vi "PerisPump_queue_single.vi"(8 "Step":string="500", 9 "Time/min":i32, 10 "First step":enum16{"forward", "backward"}(ring), 11 "Address":u8=1) -> (2 "status":dbl(slide) scale=0.0..100.0)   [LabVIEW 2023]
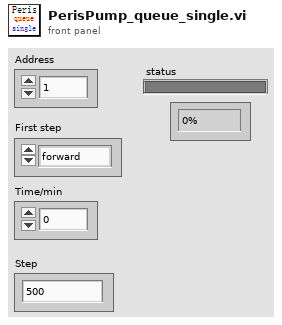
[diagram p1: front panel]
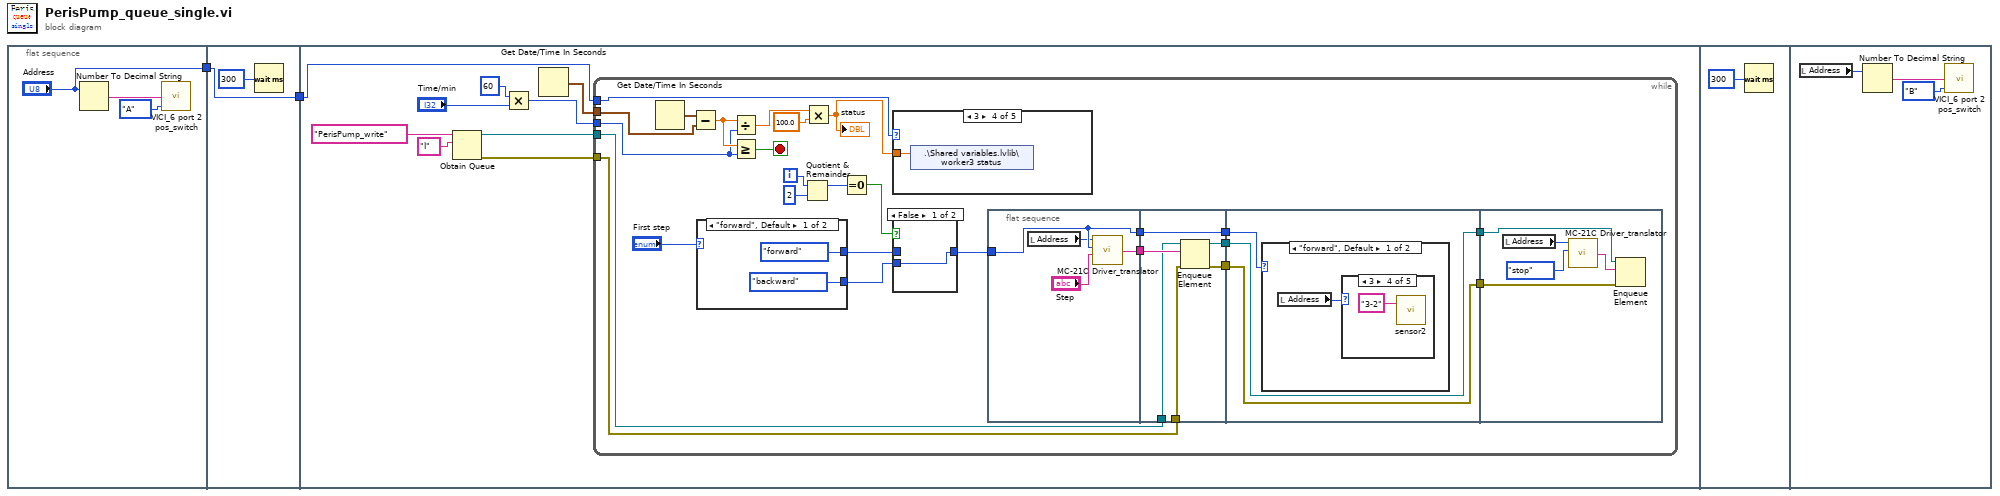
[diagram p0: block diagram]
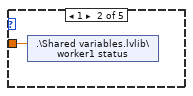
[diagram p3: hidden frame]
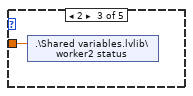
[diagram p4: hidden frame]
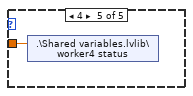
[diagram p5: hidden frame]
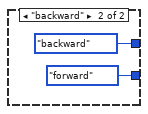
[diagram p6: hidden frame]
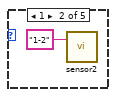
[diagram p9: hidden frame]
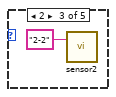
[diagram p10: hidden frame]
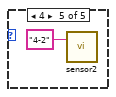
[diagram p11: hidden frame]
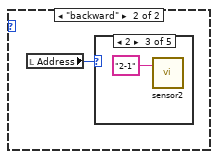
[diagram p12: hidden frame]
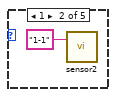
[diagram p14: hidden frame]
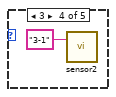
[diagram p15: hidden frame]
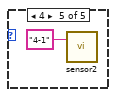
[diagram p16: hidden frame]
diagram:
  n1 = flat-sequence {
    tunnel: ["Address"] -> w1
    tunnel: [w6] -> w2
    tunnel: w1 -> [w6]
    tunnel: w2 -> [w12]
    frame #0 {
      n2 = Number To Decimal String(number="Address") -> (decimal integer string=w4:string)  [unwired: 1 in]
      n3 = call "VICI_6 port 2 pos_switch.vi"("Switch to position (A/B)"=enum16{"A", "B"}."A", "Valve ID"=w4) -> ()  [unwired: 2 in, 1 out]
    }
    frame #1 {
      n4 = Wait (ms)(milliseconds to wait=u32 300) -> ()  [unwired: 1 out]
    }
    frame #2 {
      n5 = Obtain Queue(name (unnamed)="PerisPump_write", element data type="Ì" ("string")) -> (queue out=w14:refnum<queue>, error out=w13:errorcluster)  [unwired: 3 in, 1 out]
      n6 = Multiply(x=60 ("value"), y="Time/min") -> (x*y=w8:i32)
      n7 = Get Date/Time In Seconds() -> (seconds since 1Jan1904=w11:timestamp)
      n8 = while {
        tunnel: w14 -> [w41]
        tunnel: w13 -> [w40]
        tunnel: w12 -> [w26]
        tunnel: w11 -> [w20]
        tunnel: w8 -> [w17]
        i -> [w22]
        stop <- w19 stop-if-true
        n9 = Get Date/Time In Seconds() -> (seconds since 1Jan1904=w21:timestamp)
        n10 = Subtract(x=w21, y=w20) -> (x-y=w18:dbl)
        n11 = case shown="\"forward\", Default" "First step" {
          tunnel: [enum16{"forward", "backward"}."forward" ("Operation") enum16{"forward", "backward"}."backward" ("Operation")] -> w34
          tunnel: [enum16{"forward", "backward"}."backward" ("Operation") enum16{"forward", "backward"}."forward" ("Operation")] -> w33
          frame "forward", Default {
          }
          frame "backward" {
          }
        }
        n12 = Divide(x=w18, y=w17) -> (x/y=w24:dbl)
        n13 = Greater Or Equal?(x=w18, y=w17) -> (x >= y?=w19:bool)
        n14 = Quotient & Remainder(x=w22, y=2) -> (x-y*floor(x/y)=w38:i32)  [unwired: 1 out]
        n15 = Multiply(x=w24, y=100.0) -> (x*y=w23:dbl)
        "status" <- w23
        n16 = Equal To 0?(x=w38) -> (x = 0?=w36:bool)
        n17 = case shown="3" w26 {
          tunnel: w23 -> [_ w43 w44 w45 w46]
          frame 0, Default {
          }
          frame 1 {
            n18 = shared-variable ".\\Shared variables.lvlib\\worker1 status"(w43) -> ()  [unwired: 1 in, 1 out]
          }
          frame 2 {
            n19 = shared-variable ".\\Shared variables.lvlib\\worker2 status"(w44) -> ()  [unwired: 1 in, 1 out]
          }
          frame 3 {
            n20 = shared-variable ".\\Shared variables.lvlib\\worker3 status"(w45) -> ()  [unwired: 1 in, 1 out]
          }
          frame 4 {
            n21 = shared-variable ".\\Shared variables.lvlib\\worker4 status"(w46) -> ()  [unwired: 1 in, 1 out]
          }
        }
        n22 = case shown="False" w36 {
          tunnel: [w51 w52] -> w39
          tunnel: w34 -> [_ w52]
          tunnel: w33 -> [w51 _]
          frame False {
          }
          frame True {
          }
        }
        n23 = flat-sequence {
          tunnel: [w55] -> w42
          tunnel: w39 -> [w54]
          tunnel: [w54] -> w27
          tunnel: w42 -> [w62]
          tunnel: w41 -> [w61]
          tunnel: w40 -> [w60]
          tunnel: [w59] -> w32
          tunnel: [w58] -> w29
          tunnel: [w57] -> w28
          tunnel: w27 -> [w57]
          tunnel: w32 -> [w65]
          tunnel: [w65] -> w31
          tunnel: [w64] -> w30
          tunnel: w29 -> [w64]
          tunnel: w28 -> [w63]
          tunnel: w31 -> [w77]
          tunnel: w30 -> [w78]
          frame #0 {
            n24 = local read "Address"() -> (w53:u8)
            n25 = call "MC-21C Driver_translator.vi"("Step"="Step", "Operation"=w54, "Address"=w53) -> ("Write buffer"=w55:string)  [unwired: 3 in]
          }
          frame #1 {
            n26 = Enqueue Element(queue=w61, element=w62, error in (no error)=w60) -> (queue out=w58:refnum<queue>, error out=w59:errorcluster)  [unwired: 1 in, 1 out]
          }
          frame #2 {
            n27 = case shown="\"forward\", Default" w63 {
              frame "forward", Default {
                n28 = local read "Address"() -> (w66:u8)
                n29 = case shown="3" w66 {
                  frame 0, Default {
                  }
                  frame 1 {
                    n30 = call "sensor2.vi"("Sensor"="1-2") -> ()  [unwired: 1 in, 2 out]
                  }
                  frame 2 {
                    n31 = call "sensor2.vi"("Sensor"="2-2") -> ()  [unwired: 1 in, 2 out]
                  }
                  frame 3 {
                    n32 = call "sensor2.vi"("Sensor"="3-2") -> ()  [unwired: 1 in, 2 out]
                  }
                  frame 4 {
                    n33 = call "sensor2.vi"("Sensor"="4-2") -> ()  [unwired: 1 in, 2 out]
                  }
                }
              }
              frame "backward" {
                n34 = local read "Address"() -> (w71:u8)
                n35 = case shown="2" w71 {
                  frame 0, Default {
                  }
                  frame 1 {
                    n36 = call "sensor2.vi"("Sensor"="1-1") -> ()  [unwired: 1 in, 2 out]
                  }
                  frame 2 {
                    n37 = call "sensor2.vi"("Sensor"="2-1") -> ()  [unwired: 1 in, 2 out]
                  }
                  frame 3 {
                    n38 = call "sensor2.vi"("Sensor"="3-1") -> ()  [unwired: 1 in, 2 out]
                  }
                  frame 4 {
                    n39 = call "sensor2.vi"("Sensor"="4-1") -> ()  [unwired: 1 in, 2 out]
                  }
                }
              }
            }
          }
          frame #3 {
            n40 = local read "Address"() -> (w76:u8)
            n41 = call "MC-21C Driver_translator.vi"("Operation"=enum16{"forward", "backward", "stop"}."stop", "Address"=w76) -> ("Write buffer"=w79:string)  [unwired: 4 in]
            n42 = Enqueue Element(queue=w78, element=w79, error in (no error)=w77) -> ()  [unwired: 1 in, 3 out]
          }
        }
      }
    }
    frame #3 {
      n43 = Wait (ms)(milliseconds to wait=u32 300) -> ()  [unwired: 1 out]
    }
    frame #4 {
      n44 = local read "Address"() -> (w82:u8)
      n45 = Number To Decimal String(number=w82) -> (decimal integer string=w84:string)  [unwired: 1 in]
      n46 = call "VICI_6 port 2 pos_switch.vi"("Switch to position (A/B)"=enum16{"A", "B"}."B", "Valve ID"=w84) -> ()  [unwired: 2 in, 1 out]
    }
  }
